vi "Serialize to JSON.vi"(8 "error in":errorcluster, 11 "CVT Session In":T1) -> (0 "error out":errorcluster, 2 "SerializedString":string, 3 "CVT Session Out":T1)   [LabVIEW 2015, in "CVT.lvclass"]
uses:
  CVT.lvclass
  _Session Fwk/Typedefs/Session Handle.ctl
  _Session Fwk/Session - Root.lvclass
  CVT.lvclass/CVT.ctl
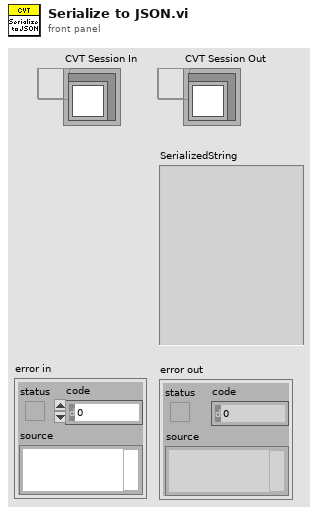
[diagram p1: front panel]
types:
  T1 = typedef "Session - Root.lvclass/Session Handle.ctl" = refnum<data-value>
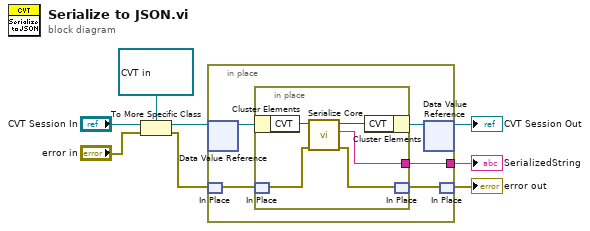
[diagram p0: block diagram]
diagram:
  n1 = To More Specific Class(target class=refnum<data-value> refnum, reference="CVT Session In", error in="error in") -> (specific class reference=w5:refnum<data-value>, error out=w2:errorcluster)
  n2 = in-place {
    in-place-border: [w11] -> w4
    n3 = in-place-dvr #1(w5) -> (w13:refnum<class "CVT.lvclass">)  [unwired: 1 out]
    n4 = in-place-match #2(w2) -> (w10:errorcluster)
    n5 = in-place {
      in-place-border: [w16] -> w11
      n6 = in-place-cluster #3(w13) -> ("CVT"=w18:variant)
      n7 = in-place-match #4(w10) -> (w15:errorcluster)
      n8 = call "Serialize Core.vi"("error in"=w15, "variant"=w18) -> ("error out"=w14:errorcluster, "StrOut"=w16:string, "Variant"=w17:variant)  [unwired: 6 in, 1 out]
      n9 = in-place-cluster #3("CVT"=w17) -> (w12:refnum<class "CVT.lvclass">)
      n10 = in-place-match #4(w14) -> (w9:errorcluster)
    }
    n11 = in-place-dvr #1(w12) -> (→"CVT Session Out":refnum<data-value>)  [unwired: 1 out]
    n12 = in-place-match #2(w9) -> (→"error out":errorcluster)
  }
  "SerializedString" <- w4
